vi "Initialize.vi"(8 "error in (no error)":errorcluster, 9 "Reset (True)":bool=TRUE, 10 "ID Query (True)":bool=TRUE, 11 "VISA resource name":refnum<visa-resource-name>) -> (0 "error out":errorcluster, 3 "VISA resource name out":refnum<visa-resource-name>)   [LabVIEW 2017, in "Keithley 2450.lvlib"]
doc: "Establishes communication with the instrument and optionally performs an instrument identification query and/or an instrument reset. It also places the instrument in a default state needed for other instrument driver operations. Therefore, call this VI before calling other instrument driver VIs for this instrument. Generally, you need to call the Initialize VI only once at the beginning of an application."
uses:
  Keithley 2450.lvlib
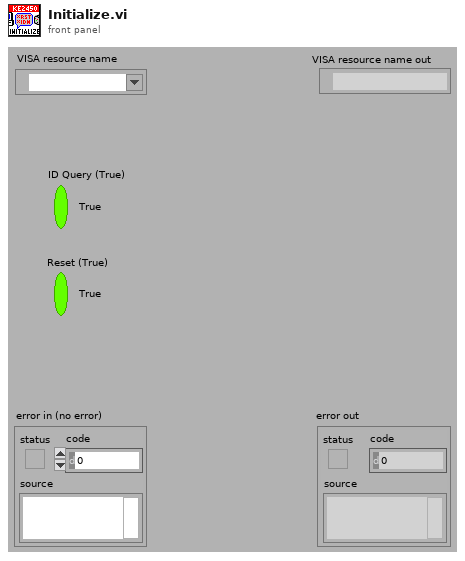
[diagram p1: front panel]
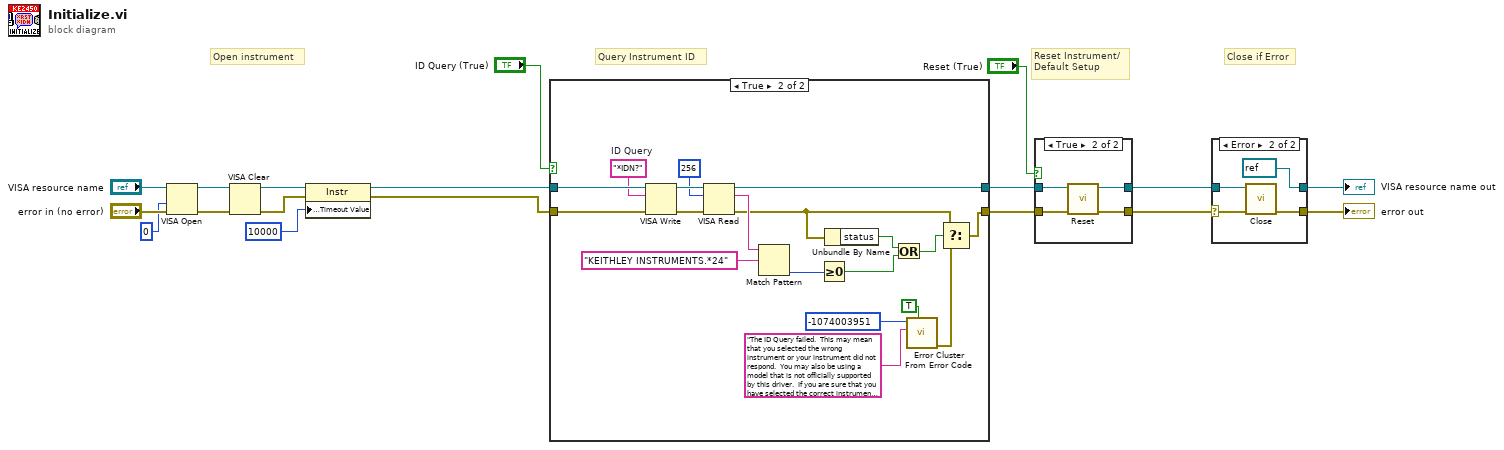
[diagram p0: block diagram]
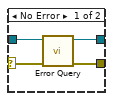
[diagram p2: hidden frame]
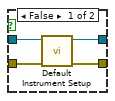
[diagram p3: hidden frame]
diagram:
  # "Close if Error"
  # "Query Instrument ID"
  # "Reset Instrument/\nDefault Setup"
  # "Open instrument"
  n1 = VISA Open(access mode=u32 0, error in (no error)="error in (no error)", VISA resource name="VISA resource name") -> (VISA resource name=w8:refnum<visa-resource-name>, error out=w7:errorcluster)  [unwired: 2 out]
  n2 = VISA Clear(VISA resource name=w8, error in (no error)=w7) -> (VISA resource name out=w6:refnum<visa-resource-name>, error out=w5:errorcluster)
  n3 = property class="Instr"(reference=w6, error in=w5, "General Settings:Timeout Value"=u32 10000) -> (reference out=w11:refnum<visa-resource-name>, error out=w10:errorcluster)
  n4 = case shown="True" "ID Query (True)" {
    tunnel: [w19 w39] -> w17
    tunnel: [w20 w36] -> w18
    tunnel: w11 -> [w20 w37]
    tunnel: w10 -> [w19 w38]
    frame False {
    }
    frame True {
      w30 = "*IDN?"  # ID Query
      n5 = VISA Write(VISA resource name=w37, write buffer=w30, error in (no error)=w38) -> (VISA resource name out=w34:refnum<visa-resource-name>, error out=w33:errorcluster)  [unwired: 1 out]
      n6 = VISA Read(VISA resource name=w34, byte count=u32 256, error in (no error)=w33) -> (VISA resource name out=w36:refnum<visa-resource-name>, read buffer=w35:string, error out=w24:errorcluster)  [unwired: 1 out]
      n7 = Match Pattern(string=w35, regular expression="KEITHLEY INSTRUMENTS.*24") -> (offset past match=w25:i32)  [unwired: 4 out]
      n8 = Greater Or Equal To 0?(x=w25) -> (x >= 0?=w22:bool)
      n9 = Unbundle By Name(w24) -> ("status"=w23:bool)
      n10 = Or(x=w23, y=w22) -> (x .or. y?=w21:bool)
      n11 = call <vilib>:"Error Cluster From Error Code.vi"("show call chain? (False)"=TRUE, "error message (\"\")"="The ID Query failed.  This may mean that you selected the wrong instrument or your instrument did not respond.  You may also be using a model that is not officially supported by this driver.  If you are sure that you have selected the correct instrument and it is responding, try disabling the ID Query." ("Source (VI Name)"), "error code (0)"=-1074003951 ("Code")) -> ("error out"=w29:errorcluster)  [unwired: 1 in, 5 out]
      n12 = Select(t=w24, s=w21, f=w29) -> (s? t:f=w39:errorcluster)
    }
  }
  n13 = case shown="True" "Reset (True)" {
    tunnel: w17 -> [w42 w44]
    tunnel: [w41 w47] -> w1
    tunnel: w18 -> [w43 w45]
    tunnel: [w40 w46] -> w2
    frame False {
      n14 = call "Default Instrument Setup.vi"("error in (no error)"=w42, "VISA resource name"=w43) -> ("error out"=w41:errorcluster, "VISA resource name out"=w40:refnum<visa-resource-name>)  [unwired: 8 out]
    }
    frame True {
      n15 = call "Reset.vi"("error in (no error)"=w44, "VISA resource name"=w45) -> ("error out"=w47:errorcluster, "VISA resource name out"=w46:refnum<visa-resource-name>)  [unwired: 8 out]
    }
  }
  n16 = case shown="Error" w1 {
    selector: w1 -> [w49 w53]
    tunnel: w2 -> [w48 w54]
    tunnel: [w51 refnum<visa-resource-name> refnum ("VISA resource name out")] -> w4
    tunnel: [w50 w55] -> w3
    frame No Error {
      n17 = call "Error Query.vi"("error in (no error)"=w49, "VISA resource name"=w48) -> ("error out"=w50:errorcluster, "VISA resource name out"=w51:refnum<visa-resource-name>)  [unwired: 8 out]
    }
    frame Error {
      n18 = call "Close.vi"("error in (no error)"=w53, "VISA resource name"=w54) -> ("error out"=w55:errorcluster)  [unwired: 9 out]
    }
  }
  "VISA resource name out" <- w4
  "error out" <- w3
